vi "Keyboard Test.vi"() -> ()   [LabVIEW 2014]
panel:
  in  "stop":bool
  in  "Speed value":dbl=1.0
  out "Control cluster":T1 {"Roll" scale=-1.0..1.0; "Pitch" scale=-1.0..1.0; "Vertical Speed" scale=-1.0..1.0; "Yaw Speed" scale=-1.0..1.0}
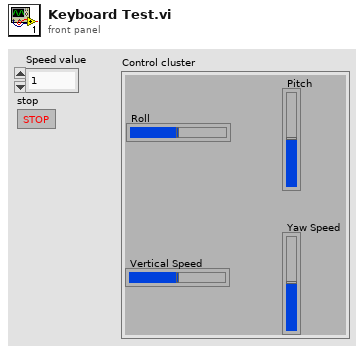
[diagram p1: front panel]
types:
  T1 = cluster{"Roll":dbl, "Pitch":dbl, "Vertical Speed":dbl, "Yaw Speed":dbl}
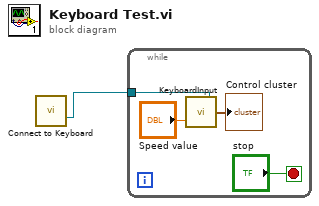
[diagram p0: block diagram]
diagram:
  n1 = call "Connect to Keyboard.vi"() -> ("device ID"=w1:refnum<k1>)  [unwired: 13 in, 2 out]
  n2 = while {
    tunnel: w1 -> [w5]
    stop <- "stop" stop-if-true
    n3 = call "KeyboardInput.vi"("Speed value"="Speed value", "device ID"=w5) -> ("Control cluster"=→"Control cluster":T1)  [unwired: 1 in, 1 out]
  }
